vi "Create_error_message.vi"(10 "Write data parameters in":T1 caption="Data Storage" {"Data storage"."Detector number" format="%#.0f"}, 11 "Status/Errors in":refnum<vi>) -> (1 "Error message":cluster{"New message ?":bool, "Message":string}, 2 "Write data parameters out":T1 caption="Data Storage" {"Data storage"."Detector number" format="%#.0f"}, 3 "Status/Errors out":refnum<vi>)   [LabVIEW 2010]
uses:
  Controls/Write_Data_Parameters.ctl
  Controls/Stop_Loop.ctl
  Controls/Data_Storage.ctl
  Controls/DB_Connection.ctl
  database/Connection.llb/Conn ObjectReference.ctl
  Controls/Data_Storage_Condition.ctl
  Controls/GPS_Timestamp.ctl
  Controls/Status_Errors_Elements.ctl
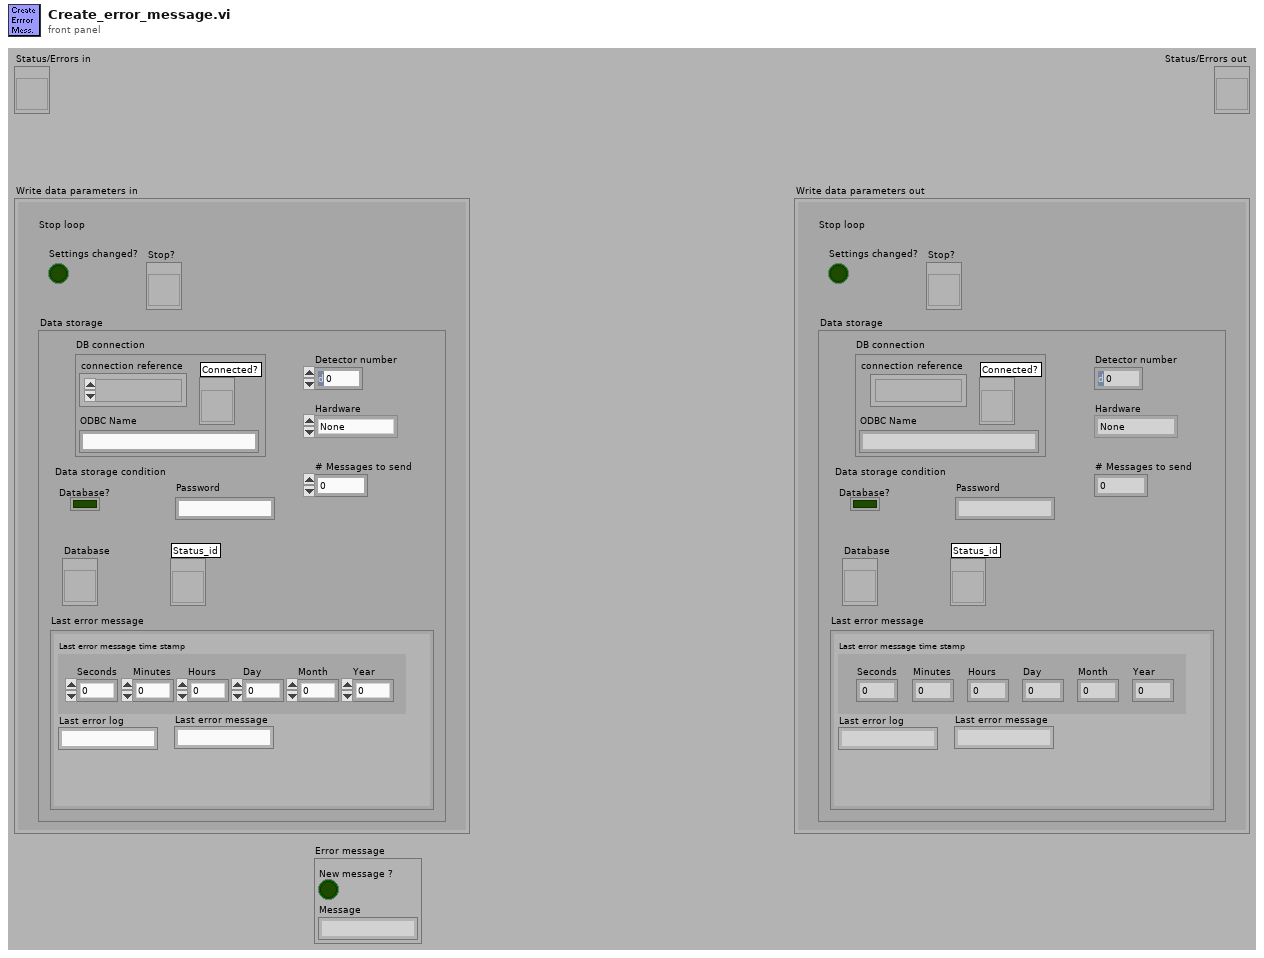
[diagram p1: front panel]
types:
  T1 = typedef "Write_Data_Parameters.ctl" = cluster{"Stop loop":T2, "Data storage":T3}
  T2 = typedef "Stop_Loop.ctl" = cluster{"Settings changed?":bool, "Stop?":refnum<vi>}
  T3 = typedef "Data_Storage.ctl" = cluster{"DB connection":T4, "Data storage condition":T6, "Detector number":u16, "# Messages to send":i32, "Database":refnum<vi>, "Password":string, "Last error message":cluster{"Last error message time stamp":T7, "Last error log":string, "Last error message":string}, "Status_id":refnum<vi>, "Hardware":enum8{"None", "HiSPARC I", "HiSPARC II", "HiSPARC III", "Unknown"}}
  T4 = typedef "DB_Connection.ctl" = cluster{"connection reference":T5, "Connected?":refnum<vi>, "ODBC Name":string}
  T5 = typedef "Conn ObjectReference.ctl" = refnum<k1>
  T6 = typedef "Data_Storage_Condition.ctl" = cluster{"Database?":bool}
  T7 = typedef "GPS_Timestamp.ctl" = cluster{"Seconds":u8, "Minutes":u8, "Hours":u8, "Day":u8, "Month":u8, "Year":u16}
  T8 = typedef "Status_Errors_Elements.ctl" = enum16{"Default", "Errors", "Master status", "Slave status", "Master connected?", "Slave connected?", "Master GPS on board?", "Slave GPS on board?", "Master: slave detected?", "Slave: slave detected?", "Last message from master", "Last message from slave", "Master temperature"}
  T9 = typedef "LVDateTimeRec.ctl" = cluster{"fractional second":dbl, "second":i32, "minute":i32, "hour":i32, "day of month":i32, "month":i32, "year":i32, "day of week":i32, "day of year":i32, "DST":i32}
  T10 = cluster{"Version number":u8, "Database":u8, "GPS timestamp":T7, "Error message":string}
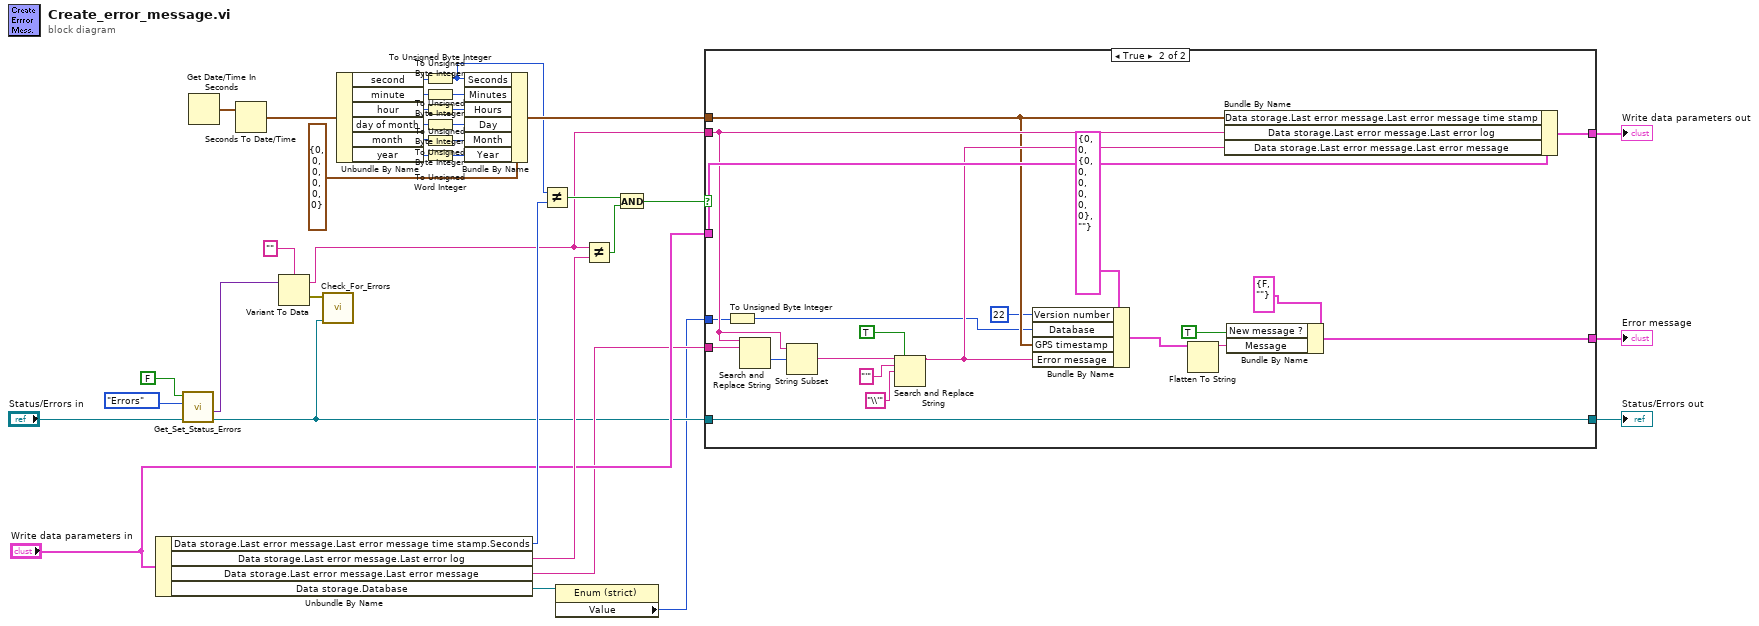
[diagram p0: block diagram]
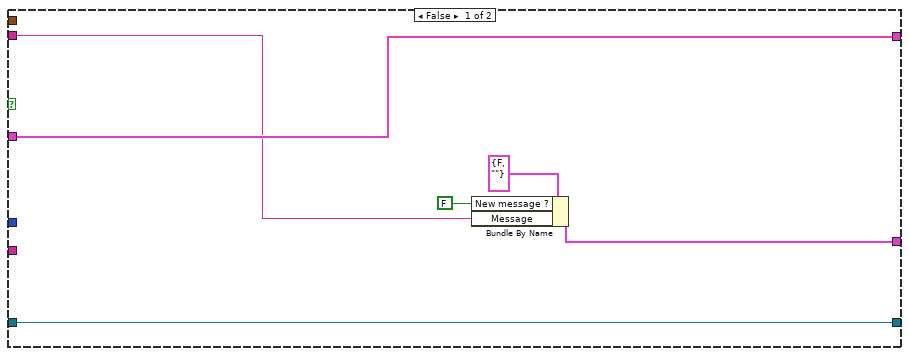
[diagram p2: hidden frame]
diagram:
  n1 = Unbundle By Name("Write data parameters in") -> ("Data storage.Last error message.Last error message time stamp.Seconds"=w22:u8, "Data storage.Last error message.Last error log"=w19:string, "Data storage.Last error message.Last error message"=w5:string, "Data storage.Database"=w2:refnum<vi>)
  n2 = call "Get_Set_Status_Errors.vi"("Status/Errors in"="Status/Errors in", "Element"=Status_Errors_Elements."Errors", "Set?"=FALSE) -> ("Status/Errors out"=w4:refnum<vi>, "Value out"=w33:variant)  [unwired: 1 in, 6 out]
  n3 = Get Date/Time In Seconds() -> (seconds since 1Jan1904=w32:timestamp)
  n4 = Seconds To Date/Time(time stamp (now)=w32) -> (date time rec=w31:T9)  [unwired: 1 out]
  n5 = Variant To Data(Variant=w33, type="") -> (error out=w12:errorcluster, data=w10:string)  [unwired: 1 in]
  n6 = call "Check_For_Errors.vi"("Status/Errors in"=w4, "error in"=w12) -> ()  [unwired: 10 out]
  n7 = Unbundle By Name(w31) -> ("second"=w30:i32, "minute"=w26:i32, "hour"=w27:i32, "day of month"=w28:i32, "month"=w29:i32, "year"=w24:i32)
  n8 = To Unsigned Byte Integer(number=w30) -> (unsigned 8bit integer=w6:u8)
  n9 = To Unsigned Byte Integer(number=w26) -> (unsigned 8bit integer=w8:u8)
  n10 = To Unsigned Byte Integer(number=w27) -> (unsigned 8bit integer=w7:u8)
  n11 = To Unsigned Byte Integer(number=w28) -> (unsigned 8bit integer=w25:u8)
  n12 = To Unsigned Byte Integer(number=w29) -> (unsigned 8bit integer=w16:u8)
  n13 = To Unsigned Word Integer(number=w24) -> (unsigned 16bit integer=w21:u16)
  n14 = Bundle By Name(cluster=T7 {"Seconds"=0, "Minutes"=0, "Hours"=0, "Day"=0, "Month"=0, "Year"=0} ("Last error message.Last error message time stamp"), "Seconds"=w6, "Minutes"=w8, "Hours"=w7, "Day"=w25, "Month"=w16, "Year"=w21) -> (w15:T7)
  n15 = Not Equal?(x=w6, y=w22) -> (x != y?=w20:bool)
  n16 = property class="Enum (strict)"(reference=w2) -> ("Value"=w1:enum8{"none", "local", "central", "both"})  [unwired: 1 in, 2 out]
  n17 = Not Equal?(x=w10, y=w19) -> (x != y?=w18:bool)
  n18 = And(x=w20, y=w18) -> (x .and. y?=w9:bool)
  n19 = case shown="True" w9 {
    tunnel: w10 -> [w39 w56]
    tunnel: "Write data parameters in" -> [w42 w63]
    tunnel: w15 -> [_ w46]
    tunnel: [w42 w62] -> w14
    tunnel: [w40 w61] -> w13
    tunnel: w5 -> [_ w58]
    tunnel: w4 -> [w37 w52]
    tunnel: [w37 w52] -> w3
    tunnel: w1 -> [_ w44]
    frame False {
      n20 = Bundle By Name(cluster=cluster{"New message ?":bool, "Message":string} {"New message ?"=FALSE, "Message"=""} ("Error message"), "New message ?"=FALSE, "Message"=w39) -> (w40:cluster{"New message ?":bool, "Message":string})
    }
    frame True {
      n21 = To Unsigned Byte Integer(number=w44) -> (unsigned 8bit integer=w43:u8)
      n22 = Search and Replace String(input string=w56, search string=w58) -> (offset past replacement=w57:i32)  [unwired: 1 in, 8 out]
      n23 = String Subset(string=w56, offset (0)=w57) -> (substring=w48:string)  [unwired: 1 out]
      n24 = Search and Replace String(replace all?=TRUE ("replace all? (F)"), input string=w48, search string="'", replace string="\\'" ("replace string (\"\")")) -> (result string=w47:string)  [unwired: 1 in, 6 out]
      n25 = Bundle By Name(cluster=T10 {"Version number"=0, "Database"=0, "GPS timestamp"={"Seconds"=0, "Minutes"=0, "Hours"=0, "Day"=0, "Month"=0, "Year"=0}, "Error message"=""} ("Cluster"), "Version number"=u8 22, "Database"=w43, "GPS timestamp"=w46, "Error message"=w47) -> (w55:T10)
      n26 = Flatten To String(anything=w55) -> (data string=w53:string)  [unwired: 1 in, 4 out]
      n27 = Bundle By Name(cluster=w63, "Data storage.Last error message.Last error message time stamp"=w46, "Data storage.Last error message.Last error log"=w56, "Data storage.Last error message.Last error message"=w47) -> (w62:T1)
      n28 = Bundle By Name(cluster=cluster{"New message ?":bool, "Message":string} {"New message ?"=FALSE, "Message"=""} ("Error message"), "New message ?"=TRUE, "Message"=w53) -> (w61:cluster{"New message ?":bool, "Message":string})
    }
  }
  "Status/Errors out" <- w3
  "Write data parameters out" <- w14
  "Error message" <- w13
